vi "Check for Job Ready.vi"(4 "File Count":i32=2, 5 "First Call?":bool, 6 "error in":errorcluster, 8 "New Jobs":string[](array[string]), 9 "Input Buffer":path) -> (0 "error out":errorcluster, 2 "Ready Jobs":string[](array[string]), 3 "Input Buffer Out":path)   [LabVIEW 2015]
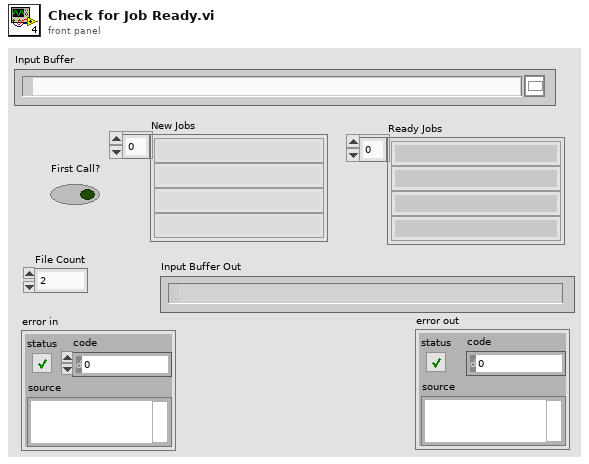
[diagram p1: front panel]
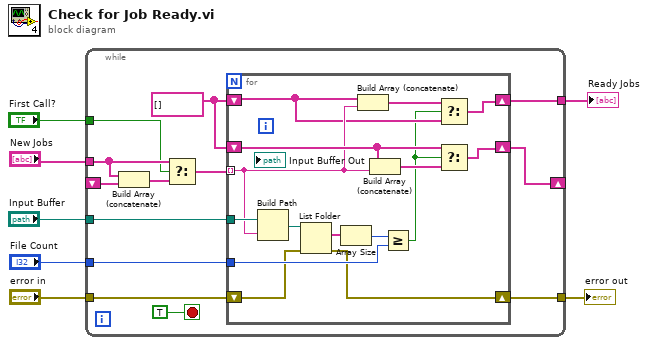
[diagram p0: block diagram]
diagram:
  n1 = while {
    shift-right: [w10] -> _
    shift-left: _ -> [w16]
    tunnel: "Input Buffer" -> [w20]
    tunnel: "File Count" -> [w18]
    tunnel: "New Jobs" -> [w14]
    tunnel: "First Call?" -> [w13]
    tunnel: [w11] -> w3
    tunnel: "error in" -> [w9]
    tunnel: [w8] -> w1
    stop <- TRUE stop-if-true
    w12 = string[] []
    n2 = Build Array (concatenate)(w14, w16) -> (w15:string[])
    n3 = Select(t=w14, s=w13, f=w15) -> (s? t:f=w17:string[])
    n4 = for {
      tunnel: w20 -> [w35]
      tunnel: w17 -> [w27] mode=indexing
      tunnel: w18 -> [w31]
      shift-right: [w24] -> w11
      shift-left: w12 -> [w25]
      shift-right: [w28] -> w10
      shift-left: w12 -> [w29]
      shift-right: [w21] -> w8
      shift-left: w9 -> [w22]
      n5 = Build Path(base path=w35, name or relative path=w27) -> (appended path=w34:path)
      n6 = List Folder(path=w34, error in=w22) -> (filenames=w33:string[], error out=w21:errorcluster)  [unwired: 2 in, 2 out]
      n7 = Array Size(array=w33) -> (size(s)=w32:i32)
      n8 = Build Array (concatenate)(w25, w27) -> (w26:string[])
      n9 = Build Array (concatenate)(w29, w27) -> (w30:string[])
      n10 = Greater Or Equal?(x=w32, y=w31) -> (x >= y?=w23:bool)
      n11 = Select(t=w26, s=w23, f=w25) -> (s? t:f=w24:string[])
      n12 = Select(t=w29, s=w23, f=w30) -> (s? t:f=w28:string[])
    }
  }
  "error out" <- w1
  "Ready Jobs" <- w3
